vi "factorial_while.vi"() -> ()   [LabVIEW 2015]
panel:
  out "Numeric 2":i32
  in  "Numeric":i32
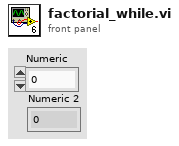
[diagram p1: front panel]
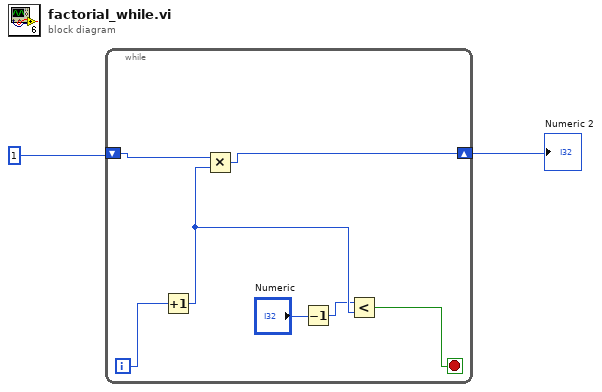
[diagram p0: block diagram]
diagram:
  n1 = while {
    shift-right: [w7] -> w1
    shift-left: 1 -> [w8]
    i -> [w9]
    stop <- w6 stop-if-true
    n2 = Increment(x=w9) -> (x+1=w5:i32)
    n3 = Multiply(x=w8, y=w5) -> (x*y=w7:i32)
    n4 = Decrement(x="Numeric") -> (x-1=w3:i32)
    n5 = Less?(x=w3, y=w5) -> (x < y?=w6:bool)
  }
  "Numeric 2" <- w1
